vi "Main_gyro.vi"() -> ()   [LabVIEW 2015]
uses:
  <vilib>/myRIO/Instrument Drivers/Onboard IO/I2C/typedefs/I2C User Configuration.ctl
  <vilib>/myRIO/Instrument Drivers/Onboard IO/I2C/typedefs/I2C Transfer Rate.ctl
  <vilib>/Platform/TimedLoop/XDataNode/timing_clust.ctl
  <vilib>/Platform/TimedLoop/XDataNode/nitl_modes.ctl
  <vilib>/Platform/TimedLoop/XDataNode/wakeup.ctl
  <vilib>/myRIO/Instrument Drivers/Onboard Devices/Accelerometer/typedefs/Accelerometer Reference.ctl
  <vilib>/myRIO/Common/Instrument Driver Framework/Utilities/typedefs/myRIO Generic Hardware Reference.ctl
  <vilib>/myRIO/Common/Instrument Driver Framework/Utilities/typedefs/Hardware Version Enum.ctl
  <vilib>/myRIO/Common/Instrument Driver Framework/Utilities/typedefs/myRIO v1.0 Reference.ctl
  <vilib>/myRIO/Common/Instrument Driver Framework/Utilities/typedefs/Generic FPGA Reference.ctl
  <vilib>/myRIO/Common/Instrument Driver Framework/myRIO v1.0/Accelerometer/typedefs/Accelerometer Channels List.ctl
  <vilib>/myRIO/Common/Instrument Driver Framework/myRIO v1.0/Accelerometer/typedefs/Accelerometer Channels Enum.ctl
  <vilib>/userdefined/High Color/nirio_resource_hc.ctl
  <vilib>/myRIO/Common/Instrument Driver Framework/Utilities/vis/Is FPGA Ref Available.vi
  <vilib>/myRIO/Common/Instrument Driver Framework/myRIO v1.0/Accelerometer/vis/myRIO v1.1 Open Accelerometer.vi
  <vilib>/myRIO/Common/Instrument Driver Framework/myRIO v1.0/DIO/vis/myRIO v1.1 Open DIO.vi
  <vilib>/myRIO/Common/Instrument Driver Framework/myRIO v1.0/I2C/vis/myRIO v1.1 Open I2C.vi
  <vilib>/myRIO/Common/Instrument Driver Framework/Utilities/vis/Validate Channels.vi
  <vilib>/myRIO/Common/Instrument Driver Framework/myRIO v1.0/Accelerometer/vis/myRIO v1.0 Reserve Accelerometer.vi
  <vilib>/myRIO/Common/Instrument Driver Framework/myRIO v1.0/UART/vis/myRIO v1.0 Close UART.vi
  <vilib>/myRIO/Common/Instrument Driver Framework/myRIO v1.0/DIO/vis/myRIO v1.0 Reserve DIO.vi
  <vilib>/myRIO/Common/Instrument Driver Framework/myRIO v1.0/I2C/vis/myRIO v1.0 Reserve I2C.vi
  <vilib>/myRIO/Common/Instrument Driver Framework/myRIO v1.0/Resource Manager/vis/myRIO v1.0 Reserve Channel List.vi
  <vilib>/myRIO/Common/Instrument Driver Framework/myRIO v1.0/Accelerometer/vis/myRIO v1.0 Build MUX Configuration Accelerometer.vi
  <vilib>/myRIO/Common/Instrument Driver Framework/myRIO v1.0/DIO/vis/myRIO v1.0 Build MUX Configuration DIO.vi
  <vilib>/myRIO/Common/Instrument Driver Framework/myRIO v1.0/I2C/vis/myRIO v1.0 Build MUX Configuration I2C.vi
  <vilib>/myRIO/Common/Instrument Driver Framework/myRIO v1.0/Resource Manager/vis/myRIO v1.0 Reserve Channel.vi
  <vilib>/myRIO/Common/Instrument Driver Framework/myRIO v1.0/Resource Manager/vis/myRIO v1.0 Unreserve Channel.vi
  <vilib>/myRIO/Common/Instrument Driver Framework/myRIO v1.0/Resource Manager/vis/myRIO v1.0 Create Configuration List.vi
  <vilib>/myRIO/Common/Instrument Driver Framework/myRIO v1.0/Resource Manager/vis/myRIO v1.0 Build Mutex Name.vi
  <vilib>/Utility/VariantDataType/GetNumericInfo.vi
  <vilib>/Utility/error.llb/Error Cluster From Error Code.vi
  <vilib>/myRIO/Common/Instrument Driver Framework/myRIO v1.0/myRIO v1.1 Open.vi
  <vilib>/myRIO/Common/Instrument Driver Framework/Utilities/vis/IO Manager.vi
  <vilib>/myRIO/Common/Instrument Driver Framework/Utilities/vis/Configuration Manager.vi
  <vilib>/myRIO/Common/Instrument Driver Framework/myRIO v1.0/Resource Manager/vis/myRIO v1.0 Configure IO.vi
  <vilib>/myRIO/Common/Instrument Driver Framework/myRIO v1.0/myRIO v1.0 Close.vi
  <vilib>/myRIO/Common/Instrument Driver Framework/myRIO v1.0/I2C/vis/myRIO v1.0 Configure I2C.vi
  <vilib>/myRIO/Common/Instrument Driver Framework/myRIO v1.0/I2C/vis/myRIO v1.0 Write I2C.vi
  <vilib>/myRIO/Common/Instrument Driver Framework/myRIO v1.0/Accelerometer/vis/myRIO v1.0 Get Scaling Constant Accelerometer.vi
  <vilib>/myRIO/Common/Instrument Driver Framework/myRIO v1.0/Accelerometer/vis/myRIO v1.0 Read Accelerometer.vi
  <vilib>/myRIO/Common/Instrument Driver Framework/myRIO v1.0/DIO/vis/myRIO v1.0 Read DIO.vi
  <vilib>/myRIO/Common/Instrument Driver Framework/myRIO v1.0/DIO/vis/myRIO v1.0 Write DIO.vi
  <vilib>/myRIO/Common/Instrument Driver Framework/myRIO v1.0/I2C/vis/myRIO v1.0 Read I2C.vi
  <vilib>/myRIO/Common/Instrument Driver Framework/Utilities/vis/FPGA Ref Manager.vi
  <vilib>/myRIO/Common/Instrument Driver Framework/myRIO v1.0/myRIO v1.0 Reset FPGA.vi
  <vilib>/myRIO/Common/Instrument Driver Framework/myRIO v1.0/IRQ/vis/myRIO v1.0 IRQ Info FGV.vi
  <vilib>/myRIO/Common/Instrument Driver Framework/myRIO v1.0/IRQ/vis/myRIO v1.0 Timer IRQ Info FGV.vi
  <vilib>/myRIO/Common/Instrument Driver Framework/myRIO v1.0/IRQ/vis/myRIO v1.0 ISR Agent.vi
  <vilib>/platform/TimedLoop/XDataNode/XDataNode.xnode
  <vilib>/myRIO/Express VI/Onboard Devices/Accelerometer/Accelerometer Express VI.xnode
  <vilib>/myRIO/Instrument Drivers/Onboard Devices/Accelerometer/vis/myRIO Accelerometer Open.xnode
  <vilib>/myRIO/Instrument Drivers/Utilities/Utilities.lvlib
  <vilib>/myRIO/Instrument Drivers/Onboard IO/I2C/I2C.lvlib
  <vilib>/myRIO/Instrument Drivers/Onboard IO/DIO/DIO.lvlib
  <vilib>/Platform/TimedLoop/XDataNode/XDNodeRunTimeDep.lvlib
  <vilib>/ptbypt/NI_PtbyPt.lvlib
  <vilib>/myRIO/Instrument Drivers/Onboard Devices/Accelerometer/Accelerometer.lvlib
panel:
  out "dtheta_dps":dbl format="%0.2f"
  out "error out_gyro":errorcluster
  out "error out_acclr":errorcluster
  out "Acceleration 2":T1(graph)
  out "theta_deg":dbl format="%0.2f"
  out "dtheta_dps":dbl format="%0.2f"
  in  "reset integrator":bool
  out "DATA":u8[](array[numeric]) format="%02x"
  out "Z rate":i16
  out "Y rate":i16
  out "X rate":i16
  in  "[ESC]":bool
  # "Gyroscope demo"
  # "OUT_X_L"
  # "OUT_X_H"
  # "OUT_Y_L"
  # "OUT_Y_H"
  # "OUT_Z_L"
  # "OUT_Z_H"
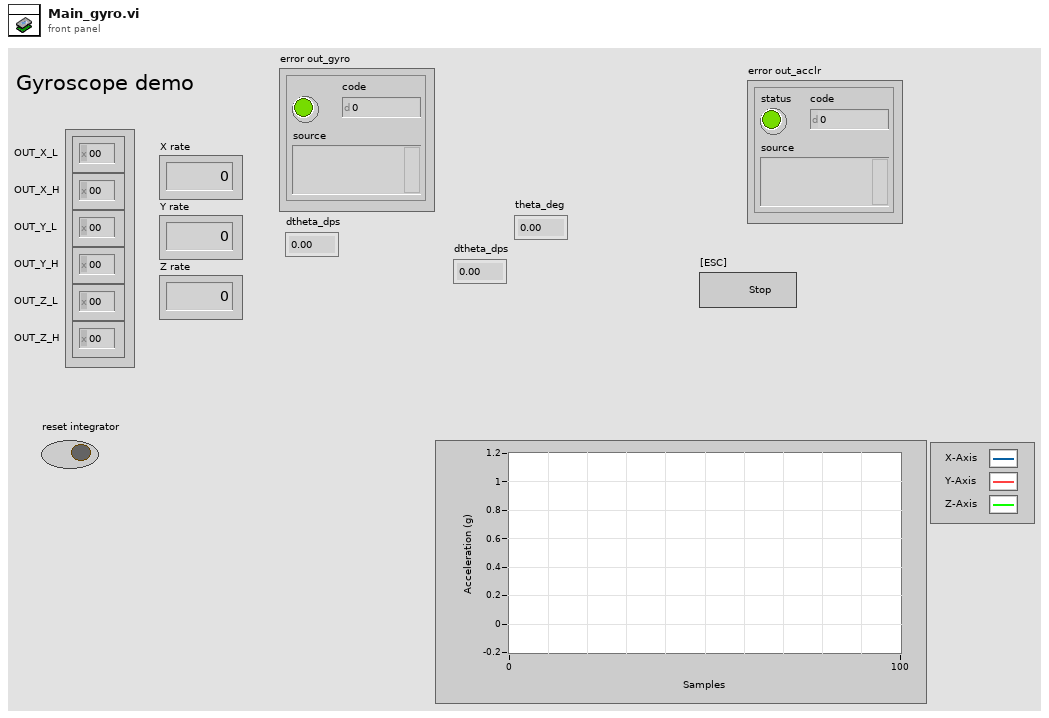
[diagram p1: front panel]
types:
  T1 = cluster{"X-Axis":dbl, "Y-Axis":dbl, "Z-Axis":dbl}
  T2 = typedef "I2C.lvlib/I2C User Configuration.ctl" = cluster{"I2C Transfer Rate":T3}
  T3 = typedef "I2C.lvlib/I2C Transfer Rate.ctl" = enum16{"Standard mode (100 kbps)", "Fast mode (400 kbps)"}
  T4 = typedef "I2C.lvlib/I2C Reference.ctl" = cluster{"myRIO Reference":T5, "I2C Channels Enum":T9, "I2C Configuration":T10}
  T5 = typedef "myRIO Generic Hardware Reference.ctl" = cluster{"myRIO Model":T6, "myRIO Hardware Reference":T7}
  T6 = typedef "Hardware Version Enum.ctl" = enum16{"Unknown", "myRIO-1900", "myRIO-1950", "roboRIO"}
  T7 = typedef "myRIO v1.0 Reference.ctl" = cluster{"Generic FPGA Reference":T8, "Allow multiple opens":bool}
  T8 = typedef "Generic FPGA Reference.ctl" = refnum<k20>
  T9 = typedef "I2C Channels Enum.ctl" = enum16{"Not Connected", "A/I2C", "B/I2C", "I2C/I2C"}
  T10 = typedef "I2C.lvlib/I2C Configuration.ctl" = cluster{"I2C Transfer Rate":T3}
  T11 = typedef "DIO.lvlib/DIO Reference.ctl" = cluster{"myRIO Reference":T5, "DIO Channels List":T12}
  T12 = typedef "DIO Channels List.ctl" = T13[]
  T13 = typedef "DIO Channels Enum.ctl" = enum16{"Not Connected", "C/DIO0", "C/DIO1", "C/DIO2", "C/DIO3", "C/DIO4", "C/DIO5", "C/DIO6", "C/DIO7", "A/DIO0", "A/DIO1", "A/DIO2", "A/DIO3", "A/DIO4", "A/DIO5", "A/DIO6", "A/DIO7", "A/DIO8", "A/DIO9", "A/DIO10", "A/DIO11", "A/DIO12", "A/DIO13", "A/DIO14", "A/DIO15", "B/DIO0", "B/DIO1", "B/DIO2", "B/DIO3", "B/DIO4", "B/DIO5", "B/DIO6", "B/DIO7", "B/DIO8", "B/DIO9", "B/DIO10", "B/DIO11", "B/DIO12", "B/DIO13", "B/DIO14", "B/DIO15", "LED0", "LED1", "LED2", "LED3", "Button0", "DIO/DIO0", "DIO/DIO1", "DIO/DIO2", "DIO/DIO3", "DIO/DIO4", "DIO/DIO5", "DIO/DIO6", "DIO/DIO7", "DIO/DIO8", "DIO/DIO9", "SPI/CS0", "SPI/CS1", "SPI/CS2", "SPI/CS3", "LED RADIO (Green)", "LED RADIO (Red)", "LED COMM (Green)", "LED COMM (Red)", "LED MODE (Green)", "LED MODE (Red)"}
  T14 = typedef "XDNodeRunTimeDep.lvlib/timing_clust.ctl" = cluster{"Expected End [f-1]":u64, "Actual End [f-1]":u64, "Finished Late? [f-1]":bool, "Expected End [i-1]":u64, "Actual End [i-1]":u64, "Finished Late? [i-1]":bool, "Expected Start [i]":u64, "Actual Start [i]":u64, "Expected Start [f]":u64, "Actual Start [f]":u64, "Source Name":string, "Structure Name":string, "Period":i64, "Deadline":i64, "Offset":i64, "Start":i64, "Priority":i32, "Timeout":i32, "Mode":T15, "Wakeup Reason":T16, "Error":errorcluster, "Source Type":string, "Secondary Source Type":string, "Global End Time":u64, "Global Start Time":u64, "Frame Duration":u64, "Iteration Duration":u64, "Assigned CPU":i32, "I/O Scan Engine Mode":u32}
  T15 = typedef "XDNodeRunTimeDep.lvlib/nitl_modes.ctl" = enum32{"No Change", "Process missed periods, maintain original phase", "Discard missed periods, maintain original phase", "Process missed periods, ignore original phase", "Discard missed periods, ignore original phase"}
  T16 = typedef "XDNodeRunTimeDep.lvlib/wakeup.ctl" = enum32{"Normal", "Aborted", "Asynchronous wakeup", "Timing source error", "Timed loop error", "Timeout"}
  T17 = typedef "Accelerometer.lvlib/Accelerometer Reference.ctl" = cluster{"myRIO Reference":T5, "Accelerometer Channels List":T18, "LSB Weight":dbl}
  T18 = typedef "Accelerometer Channels List.ctl" = T19[]
  T19 = typedef "Accelerometer Channels Enum.ctl" = enum16{"Not Connected", "X-Axis", "Y-Axis", "Z-Axis"}
  T20 = typedef "nirio_resource_hc.ctl" = tag
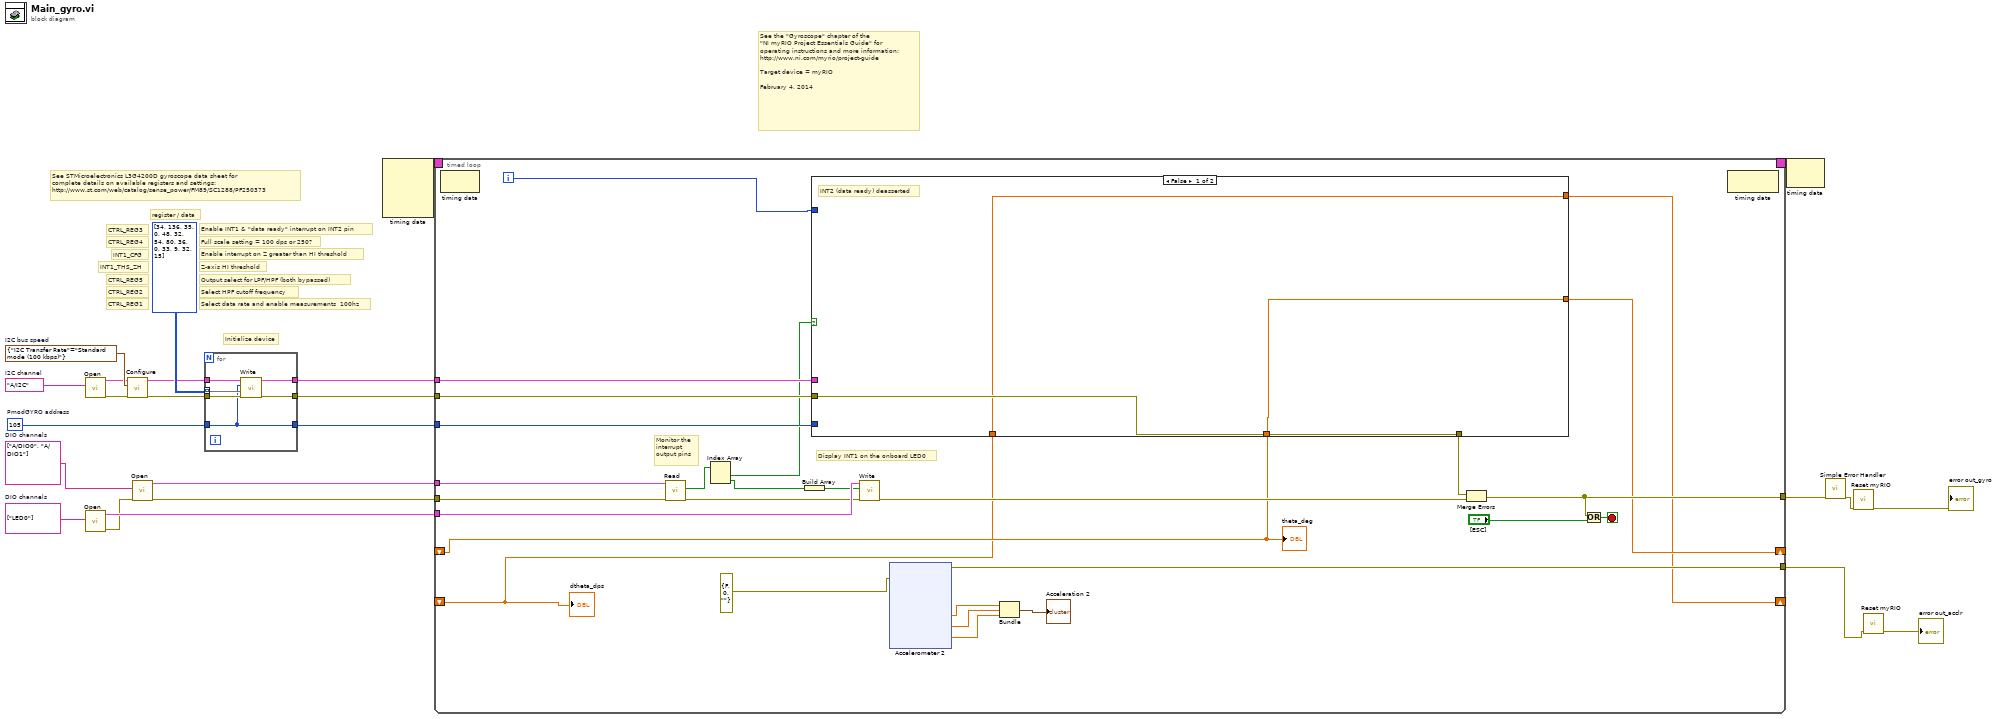
[diagram p0: block diagram]
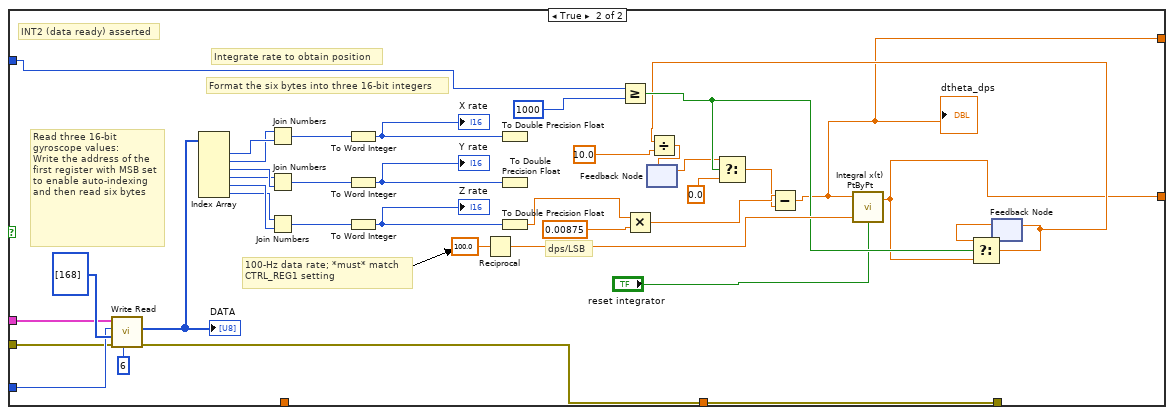
[diagram p2: hidden frame]
diagram:
  w6 = tag[] ["LED0"]  # DIO channels
  w9 = tag[] ["A/DIO0", "A/DIO1"]  # DIO channels
  w21 = T2 {"I2C Transfer Rate"=enum."Standard mode (100 kbps)"}  # I2C bus speed
  w22 = tag "A/I2C"  # I2C channel
  w12 = u8 105  # PmodGYRO address
  # "See the \"Gyroscope\" chapter of the\n\"NI myRIO Project Essentials Guide\" for\noperating instructions and more information: \nhttp://www.ni.com/myrio/project-guide\n\nTarget device = myRIO\n\nFebruary 4, 2014"
  # "Enable INT1 & \"data ready\" interrupt on INT2 pin"
  # "CTRL_REG3"
  # "Select HPF cutoff frequency"
  # "CTRL_REG2"
  # "Output select for LPF/HPF (both bypassed)"
  # "CTRL_REG5"
  # "Initialize device"
  # "Select data rate and enable measurements  100hz"
  # "Z-axis HI threshold"
  # "Enable interrupt on Z greater than HI threshold"
  # "See STMicroelectronics L3G4200D gyroscope data sheet for\ncomplete details on available registers and settings:\nhttp://www.st.com/web/catalog/sense_power/FM89/SC1288/PF250373"
  # "CTRL_REG1"
  # "INT1_THS_ZH"
  # "INT1_CFG"
  # "Full scale setting = 100 dps or 250?"
  # "CTRL_REG4"
  # "register / data"
  n1 = call <vilib>:"Open.vi"("Channel Name"=w22) -> ("error out"=w19:errorcluster, "I2C Ref Out"=w20:T4)  [unwired: 9 in]
  n2 = call <vilib>:"Open.vi"("Channel Names"=w6) -> ("error out"=w4:errorcluster, "DIO Ref Out"=w5:T11)  [unwired: 9 in]
  n3 = call <vilib>:"Configure.vi"("error in (no error)"=w19, "I2C User Configuration"=w21, "I2C Ref In"=w20) -> ("error out"=w13:errorcluster, "I2C Ref Out"=w14:T4)  [unwired: 7 in]
  n4 = call <vilib>:"Open.vi"("error in (no error)"=w4, "Channel Names"=w9) -> ("error out"=w11:errorcluster, "DIO Ref Out"=w10:T11)  [unwired: 8 in]
  n5 = for {
    tunnel: [w30] -> w18
    tunnel: [w29] -> w17
    tunnel: [w25] -> w16
    tunnel: u8[][] [[34, 136], [35, 0], [48, 32], [54, 80], [36, 0], [33, 9], [32, 15]] ("Bytes to Write") -> [w28] mode=indexing
    tunnel: w14 -> [w27]
    tunnel: w13 -> [w26]
    tunnel: w12 -> [w25]
    n6 = call <vilib>:"Write.vi"("error in (no error)"=w26, "Bytes to Write"=w28, "Slave Address (7-bit)"=w25, "I2C Ref In"=w27) -> ("error out"=w30:errorcluster, "I2C Ref Out"=w29:T4)  [unwired: 6 in]
  }
  n7 = node-c288() -> (w8:T14)  [unwired: 4 in]
  n8 = timed-loop {
    tunnel: [w42] -> w23
    tunnel: w16 -> [w53]
    tunnel: w18 -> [w55]
    tunnel: w17 -> [w54]
    tunnel: w11 -> [w52]
    tunnel: w10 -> [w51]
    timing: w8 -> [_]
    timing-out: [_] -> w7
    tunnel: w5 -> [w47]
    shift-right: [w40] -> _
    shift-left: _ -> [w39]
    tunnel: [w34] -> w2
    shift-right: [w32] -> _
    shift-left: _ -> [w31]
    i -> [w41]
    stop <- w57 stop-if-true
    # "Display INT1 on the onboard LED0"
    # "Monitor the\ninterrupt\noutput pins"
    n9 = node-c288() -> ()  [unwired: 1 in, 1 out]
    n10 = call <vilib>:"Read.vi"("error in (no error)"=w52, "DIO Ref In"=w51) -> ("error out"=w46:errorcluster, "Values"=w48:bool[])  [unwired: 7 in, 1 out]
    n11 = Index Array "Index Array"(array=w48) -> (element #1=w49:bool, element #2=w44:bool)  [unwired: 2 in]
    n12 = Build Array "Build Array"(w44) -> (w45:bool[])
    n13 = case shown="False" w49 {
      tunnel: w55 -> [w101 w120]
      tunnel: w54 -> [_ w121]
      tunnel: w53 -> [_ w127]
      tunnel: [w101 w126] -> w50
      tunnel: w41 -> [_ w106]
      tunnel: [w100 w103] -> w40
      tunnel: w39 -> [w100 _]
      tunnel: [w99 w102] -> w32
      tunnel: w31 -> [w99 _]
      frame False {
        # "INT2 (data ready) deasserted"
      }
      frame True {
        # "dps/LSB"
        # "100-Hz data rate; *must* match\nCTRL_REG1 setting"
        # "Integrate rate to obtain position"
        # "INT2 (data ready) asserted"
        # "Read three 16-bit gyroscope values:\nWrite the address of the first register with MSB set to enable auto-indexing and then read six bytes"
        # "Format the six bytes into three 16-bit integers"
        n14 = call <vilib>:"Write Read.vi"("Byte Count"=u32 6, "error in (no error)"=w120, "Bytes to Write"=u8[] [168], "Slave Address (7-bit)"=w127, "I2C Ref In"=w121) -> ("error out"=w126:errorcluster, "Bytes Read"=w125:u8[])  [unwired: 3 in, 1 out]
        "DATA" <- w125
        n15 = Index Array "Index Array"(array=w125) -> (element #1=w135:u8, element #2=w134:u8, element #3=w133:u8, element #4=w132:u8, element #5=w131:u8, element #6=w130:u8)  [unwired: 6 in]
        n16 = Join Numbers(hi=w134, lo=w135) -> ((hi.lo)=w138:u16)
        n17 = Join Numbers(hi=w132, lo=w133) -> ((hi.lo)=w137:u16)
        n18 = Join Numbers(hi=w130, lo=w131) -> ((hi.lo)=w136:u16)
        n19 = To Word Integer(number=w138) -> (16bit integer=w124:i16)
        "X rate" <- w124
        n20 = To Word Integer(number=w137) -> (16bit integer=w123:i16)
        "Y rate" <- w123
        n21 = To Word Integer(number=w136) -> (16bit integer=w122:i16)
        "Z rate" <- w122
        n22 = Reciprocal(x=100.0 ("dt")) -> (1/x=w118:dbl)
        n23 = To Double Precision Float(number=w124) -> ()  [unwired: 1 out]
        n24 = To Double Precision Float(number=w123) -> ()  [unwired: 1 out]
        n25 = To Double Precision Float(number=w122) -> (double precision float=w116:dbl)
        n26 = Greater Or Equal?(x=w106, y=1000) -> (x >= y?=w114:bool)
        n27 = Multiply(x=w116, y=0.00875) -> (x*y=w109:dbl)
        n28 = feedback #1() -> (w110:dbl)  [unwired: 1 in]
        n29 = Select(t=w110, s=w114, f=0.0) -> (s? t:f=w108:dbl)
        n30 = Subtract(x=w109, y=w108) -> (x-y=w102:dbl)
        "dtheta_dps" <- w102
        n31 = call <vilib>:"Integral x(t) PtByPt.vi"("initialize"="reset integrator", "dt"=w118, "x"=w102) -> ("integral x(t)"=w103:dbl)  [unwired: 1 in, 1 out]
        n32 = feedback #2() -> (w113:dbl)  [unwired: 1 in]
        n33 = Select(t=w113, s=w114, f=w103) -> (s? t:f=w104:dbl)
        n34 = Divide(x=w104, y=10.0 ("x")) -> (x/y=w111:dbl)
        n35 = feedback-in #1(w111) -> ()
        n36 = feedback-in #2(w104) -> ()
      }
    }
    n37 = call <vilib>:"Write.vi"("error in (no error)"=w46, "Values"=w45, "DIO Ref In"=w47) -> ("error out"=w43:errorcluster)  [unwired: 6 in, 1 out]
    n38 = xnode "Accelerometer 2"("error in (no error)"=errorcluster {"status"=FALSE, "code"=0, "source"=""}) -> ("X-Axis"=w37:dbl, "Y-Axis"=w36:dbl, "Z-Axis"=w35:dbl, "error out"=w34:errorcluster)
    n39 = Bundle("X-Axis"=w37, "Y-Axis"=w36, "Z-Axis"=w35) -> (→"Acceleration 2":T1)  [unwired: 1 in]
    n40 = Merge Errors "Merge Errors"(w50, w43) -> (w42:errorcluster)
    n41 = Or(x=w42, y="[ESC]") -> (x .or. y?=w57:bool)
    n42 = node-c288() -> ()  [unwired: 1 in, 1 out]
    "theta_deg" <- w39
    "dtheta_dps" <- w31
  }
  n43 = node-c288(w7) -> ()  [unwired: 1 out]
  n44 = call <vilib>:"Simple Error Handler.vi"("error in (no error)"=w23) -> ("error out"=w24:errorcluster)  [unwired: 4 in, 4 out]
  n45 = call <vilib>:"Reset myRIO.vi"("error in (no error)"=w24) -> ("error out"=→"error out_gyro":errorcluster)  [unwired: 10 in]
  n46 = call <vilib>:"Reset myRIO.vi"("error in (no error)"=w2) -> ("error out"=→"error out_acclr":errorcluster)  [unwired: 10 in]
